vi "VI Tree - variantconfig__lvcfg.vi"() -> ()   [LabVIEW 2017, in "LabVIEW Config(Variant).lvlib"]
uses:
  LabVIEW Config(Variant).lvlib
  <userlib>/_NEVSTOP/Communicable State Machine(CSM)/addons/INI-Static-Variable-Support/LabVIEW-Config/Config.ctl
  <userlib>/_NEVSTOP/Communicable State Machine(CSM)/addons/INI-Static-Variable-Support/LabVIEW-Config/LabVIEW-Config.lvlib
panel:
  in  "Config in":T1
  in  "VI ref":refnum<vi>
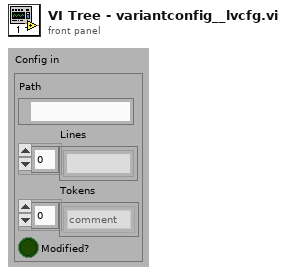
[diagram p1: front panel]
types:
  T1 = typedef "LabVIEW-Config.lvlib/Config.ctl" = cluster{"Path":path, "Lines":string[], "Tokens":enum8{"comment", "section", "key"}[], "Modified?":bool}
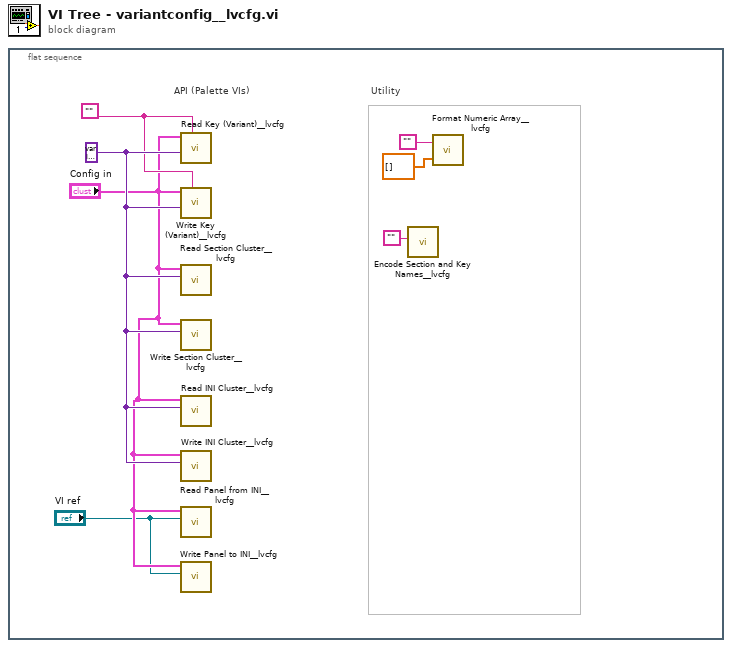
[diagram p0: block diagram]
diagram:
  n1 = flat-sequence {
    frame #0 {
      w7 = variant ("type")
      w6 = ""
      # "Utility"
      # "API (Palette VIs)"
      n2 = call "Read Key (Variant)__lvcfg.vi"("section"=w6, "type"=w7, "Config in"="Config in") -> ()  [unwired: 5 in, 4 out]
      n3 = call "Write Key (Variant)__lvcfg.vi"("section"=w6, "key-value"=w7, "Config in"="Config in") -> ()  [unwired: 7 in, 2 out]
      n4 = call "Read Section Cluster__lvcfg.vi"("Section Formatted Cluster Type"=w7, "Config in"="Config in") -> ()  [unwired: 5 in, 5 out]
      n5 = call "Write Section Cluster__lvcfg.vi"("Section Formatted Cluster"=w7, "Config in"="Config in") -> ()  [unwired: 8 in, 2 out]
      n6 = call "Read INI Cluster__lvcfg.vi"("INI Fomatted Cluster Type"=w7, "Config in"="Config in") -> ()  [unwired: 5 in, 5 out]
      n7 = call "Write INI Cluster__lvcfg.vi"("INI Fomatted Cluster"=w7, "Config out"="Config in") -> ()  [unwired: 8 in, 2 out]
      n8 = call "Read Panel from INI__lvcfg.vi"("VI ref"="VI ref", "Config out"="Config in") -> ()  [unwired: 8 in, 2 out]
      n9 = call "Write Panel to INI__lvcfg.vi"("VI ref"="VI ref", "Config out"="Config in") -> ()  [unwired: 8 in, 2 out]
      n10 = call "Encode Section and Key Names__lvcfg.vi"("string"="" ("format string")) -> ()  [unwired: 10 in, 1 out]
      n11 = call "Format Numeric Array__lvcfg.vi"("Array"=dbl[] [], "format string"="") -> ()  [unwired: 1 out]
    }
  }
